vi "stepper_setspeed.vi"(8 "error in (no error)":errorcluster, 10 "velocity parameters in":T1={"pfMinVel"=0.0, "pfAccn"=4.0, "pfMaxVel"=4.0}, 11 "reference":refnum<k7>) -> (0 "error out":errorcluster, 2 "velocity parameters out":T1={"pfMinVel"=0.0, "pfAccn"=4.0, "pfMaxVel"=4.0}, 3 "reference out":refnum<k7>)   [LabVIEW 2018]
uses:
  <userlib>/stepper/velocity settings.ctl
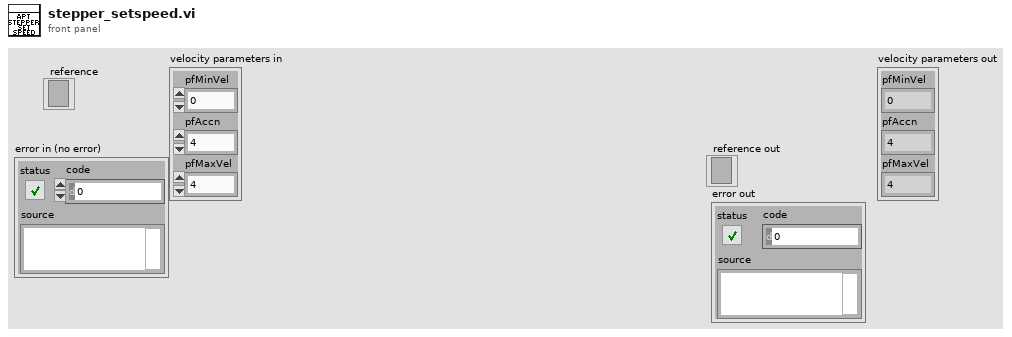
[diagram p1: front panel]
types:
  T1 = typedef "velocity settings.ctl" = cluster{"pfMinVel":sgl, "pfAccn":sgl, "pfMaxVel":sgl}
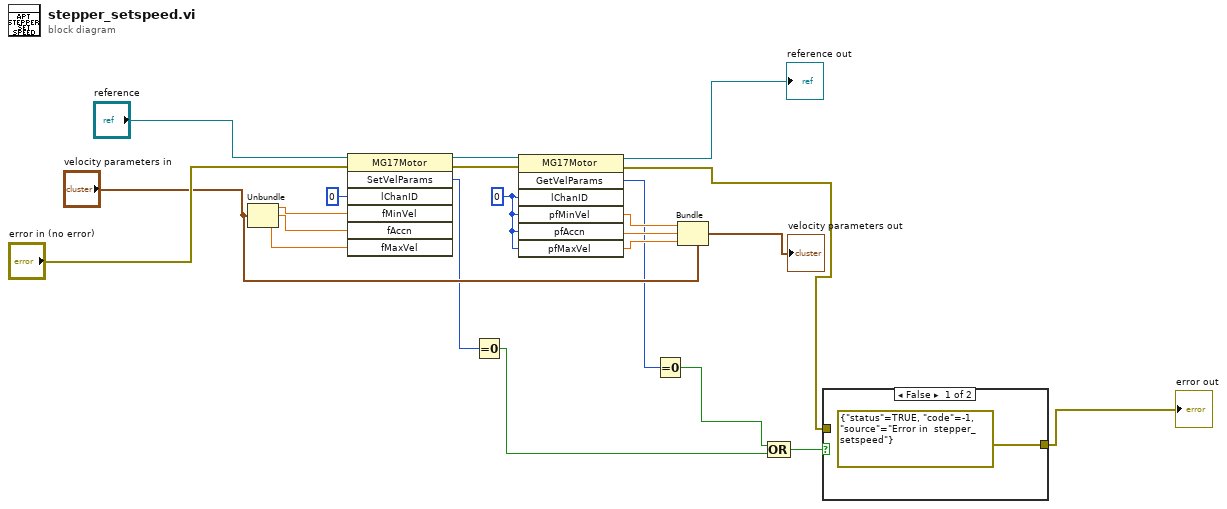
[diagram p0: block diagram]
diagram:
  w9 = 0 ("lChanID")
  n1 = Unbundle("velocity parameters in") -> ("pfMinVel"=w17:sgl, "pfAccn"=w16:sgl, "pfMaxVel"=w15:sgl)
  n2 = invoke class="MG17Motor" method="SetVelParams"(reference="reference", error in="error in (no error)", "lChanID"=0, "fMinVel"=w17, "fAccn"=w16, "fMaxVel"=w15) -> (reference out=w21:refnum<k7>, error out=w3:errorcluster, "SetVelParams"=w8:i32)  [unwired: 1 in, 4 out]
  n3 = Equal To 0?(x=w8) -> (x = 0?=w5:bool)
  n4 = invoke class="MG17Motor" method="GetVelParams"(reference=w21, error in=w3, "lChanID"=w9, "pfMinVel"=w9, "pfAccn"=w9, "pfMaxVel"=w9) -> (reference out=→"reference out":refnum<k7>, error out=w2:errorcluster, "GetVelParams"=w7:i32, "pfMinVel"=w13:sgl, "pfAccn"=w12:sgl, "pfMaxVel"=w11:sgl)  [unwired: 1 in, 1 out]
  n5 = Equal To 0?(x=w7) -> (x = 0?=w6:bool)
  n6 = Bundle(cluster="velocity parameters in", "pfMinVel"=w13, "pfAccn"=w12, "pfMaxVel"=w11) -> (→"velocity parameters out":T1)
  n7 = Compound Arithmetic op=OR(w6, w5) -> (w4:bool)
  n8 = case shown="False" w4 {
    tunnel: [errorcluster {"status"=TRUE, "code"=-1, "source"="Error in  stepper_setspeed"} ("error out") w24] -> w1
    tunnel: w2 -> [_ w24]
    frame False {
    }
    frame True {
    }
  }
  "error out" <- w1
